vi "Get Date Code.vi"() -> (0 "Day Of year":string, 3 "DateCode":string)   [LabVIEW 2017]
uses:
  <vilib>/Utility/miscctls.llb/LVDateTimeRec.ctl
panel:
  out "week":string
  in  "date time rec":T1
  out "2digitYear":string
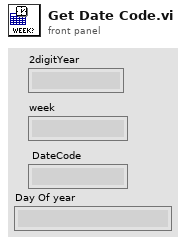
[diagram p1: front panel]
types:
  T1 = typedef "LVDateTimeRec.ctl" = cluster{"fractional second":dbl, "second":i32, "minute":i32, "hour":i32, "day of month":i32, "month":i32, "year":i32, "day of week":i32, "day of year":i32, "DST":i32}
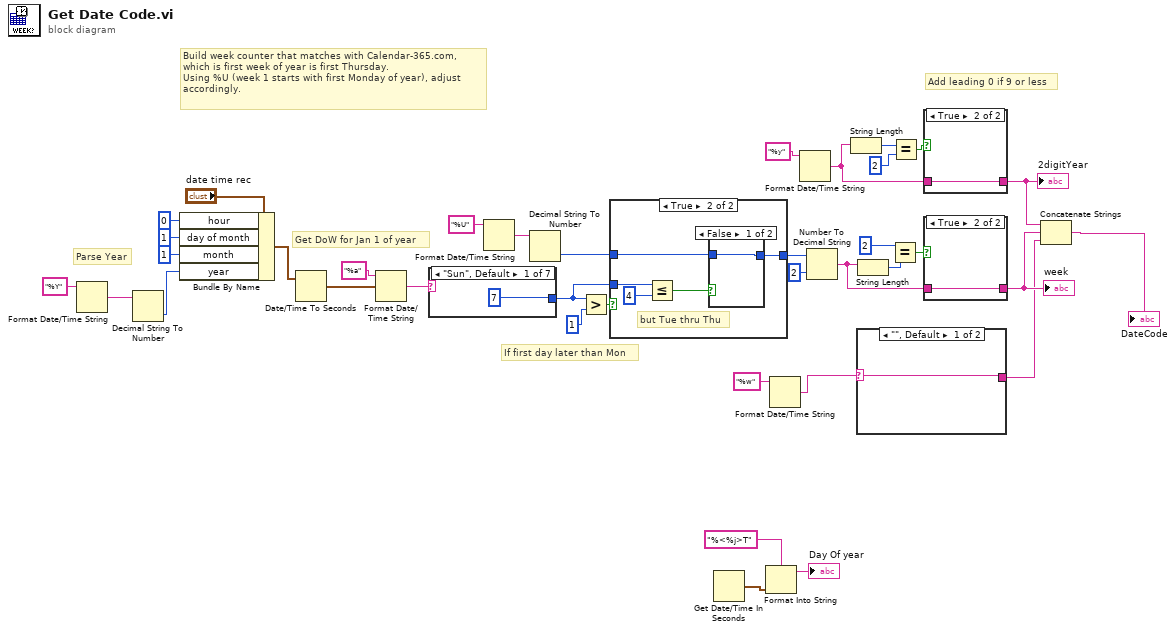
[diagram p0: block diagram]
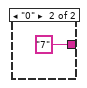
[diagram p2: hidden frame]
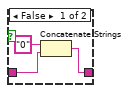
[diagram p3: hidden frame]
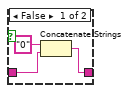
[diagram p4: hidden frame]
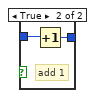
[diagram p6: hidden frame]
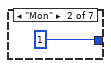
[diagram p7: hidden frame]
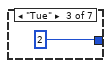
[diagram p8: hidden frame]
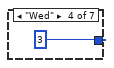
[diagram p9: hidden frame]
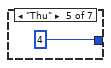
[diagram p10: hidden frame]
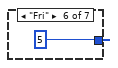
[diagram p11: hidden frame]
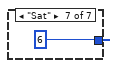
[diagram p12: hidden frame]
diagram:
  # "Add leading 0 if 9 or less"
  # "If first day later than Mon"
  # "Get DoW for Jan 1 of year"
  # "Parse Year"
  # "Build week counter that matches with Calendar-365.com,\nwhich is first week of year is first Thursday.\nUsing %U (week 1 starts with first Monday of year), adjust\naccordingly."
  n1 = Format Date/Time String(time format string (%c)="%Y") -> (date/time string=w34:string)  [unwired: 2 in]
  n2 = Decimal String To Number(string=w34) -> (number=w23:i32)  [unwired: 2 in, 1 out]
  n3 = Bundle By Name(cluster="date time rec", "hour"=0, "day of month"=1, "month"=1, "year"=w23) -> (w33:T1)
  n4 = Date/Time To Seconds(2:w33) -> (0:w9:timestamp)  [unwired: 1 in]
  n5 = Format Date/Time String(time format string (%c)="%a", seconds (now)=w9) -> (date/time string=w31:string)  [unwired: 1 in]
  n6 = case shown="\"Sun\", Default" w31 {
    tunnel: [7 1 2 3 4 5 6] -> w10
    frame "Sun", Default {
    }
    frame "Mon" {
    }
    frame "Tue" {
    }
    frame "Wed" {
    }
    frame "Thu" {
    }
    frame "Fri" {
    }
    frame "Sat" {
    }
  }
  n7 = Format Date/Time String(time format string (%c)="%U") -> (date/time string=w27:string)  [unwired: 2 in]
  n8 = Decimal String To Number(string=w27) -> (number=w26:i32)  [unwired: 2 in, 1 out]
  n9 = Greater?(x=w10, y=1) -> (0:w29:bool)
  n10 = case shown="True" w29 {
    tunnel: w10 -> [_ w50]
    tunnel: w26 -> [w45 w47]
    tunnel: [w45 w46] -> w25
    frame False {
    }
    frame True {
      # "but Tue thru Thu"
      n11 = Less Or Equal?(x=w50, y=4) -> (x <= y?=w48:bool)
      n12 = case shown="False" w48 {
        tunnel: w47 -> [w51 w53]
        tunnel: [w51 w52] -> w46
        frame False {
        }
        frame True {
          # "add 1"
          n13 = Increment(x=w53) -> (x+1=w52:i32)
        }
      }
    }
  }
  n14 = Get Date/Time In Seconds() -> (seconds since 1Jan1904=w2:timestamp)
  n15 = Format Into String(format string="%<%j>T", w2) -> (resulting string=→"Day Of year":string)  [unwired: 2 in, 1 out]
  n16 = Format Date/Time String(time format string (%c)="%w") -> (date/time string=w7:string)  [unwired: 2 in]
  n17 = Format Date/Time String(time format string (%c)="%y") -> (date/time string=w18:string)  [unwired: 2 in]
  n18 = Number To Decimal String(number=w25, width (-)=i16 2) -> (decimal integer string=w14:string)
  n19 = String Length(string=w18) -> (length=w21:i32)
  n20 = case shown="\"\", Default" w7 {
    selector: w7 -> [w54 _]
    tunnel: [w54 "7"] -> w6
    frame "", Default {
    }
    frame "0" {
    }
  }
  n21 = String Length(string=w14) -> (length=w17:i32)
  n22 = Equal?(x=2, y=w17) -> (x = y?=w15:bool)
  n23 = Equal?(x=w21, y=2) -> (x = y?=w19:bool)
  n24 = case shown="True" w19 {
    tunnel: w18 -> [w56 w59]
    tunnel: [w58 w59] -> w13
    frame False {
      n25 = Concatenate Strings("0" ("string"), w56) -> (w58:string)
    }
    frame True {
    }
  }
  "2digitYear" <- w13
  n26 = case shown="True" w15 {
    tunnel: w14 -> [w60 w63]
    tunnel: [w62 w63] -> w12
    frame False {
      n27 = Concatenate Strings("0" ("string"), w60) -> (w62:string)
    }
    frame True {
    }
  }
  "week" <- w12
  n28 = Concatenate Strings(w13, w12, w6) -> (→"DateCode":string)
